vi "Plot update numeric array.vi"(8 "error in (no error)":errorcluster, 9 "Numerics":dbl[](array[numeric]), 11 "refs":T1) -> (0 "error out":errorcluster)   [LabVIEW 2021, in "RocketPlot.lvlib"]
uses:
  RocketPlot.lvlib
  TypeDefs/Plot UI references.ctl
  Classes/RocketPlotHandle/RocketPlotHandle.lvclass
  <userlib>/bjustice/TipStripOOPanel/Classes/TipPanelHandle/TipPanelHandle.lvclass
  TypeDefs/Plot top row.ctl
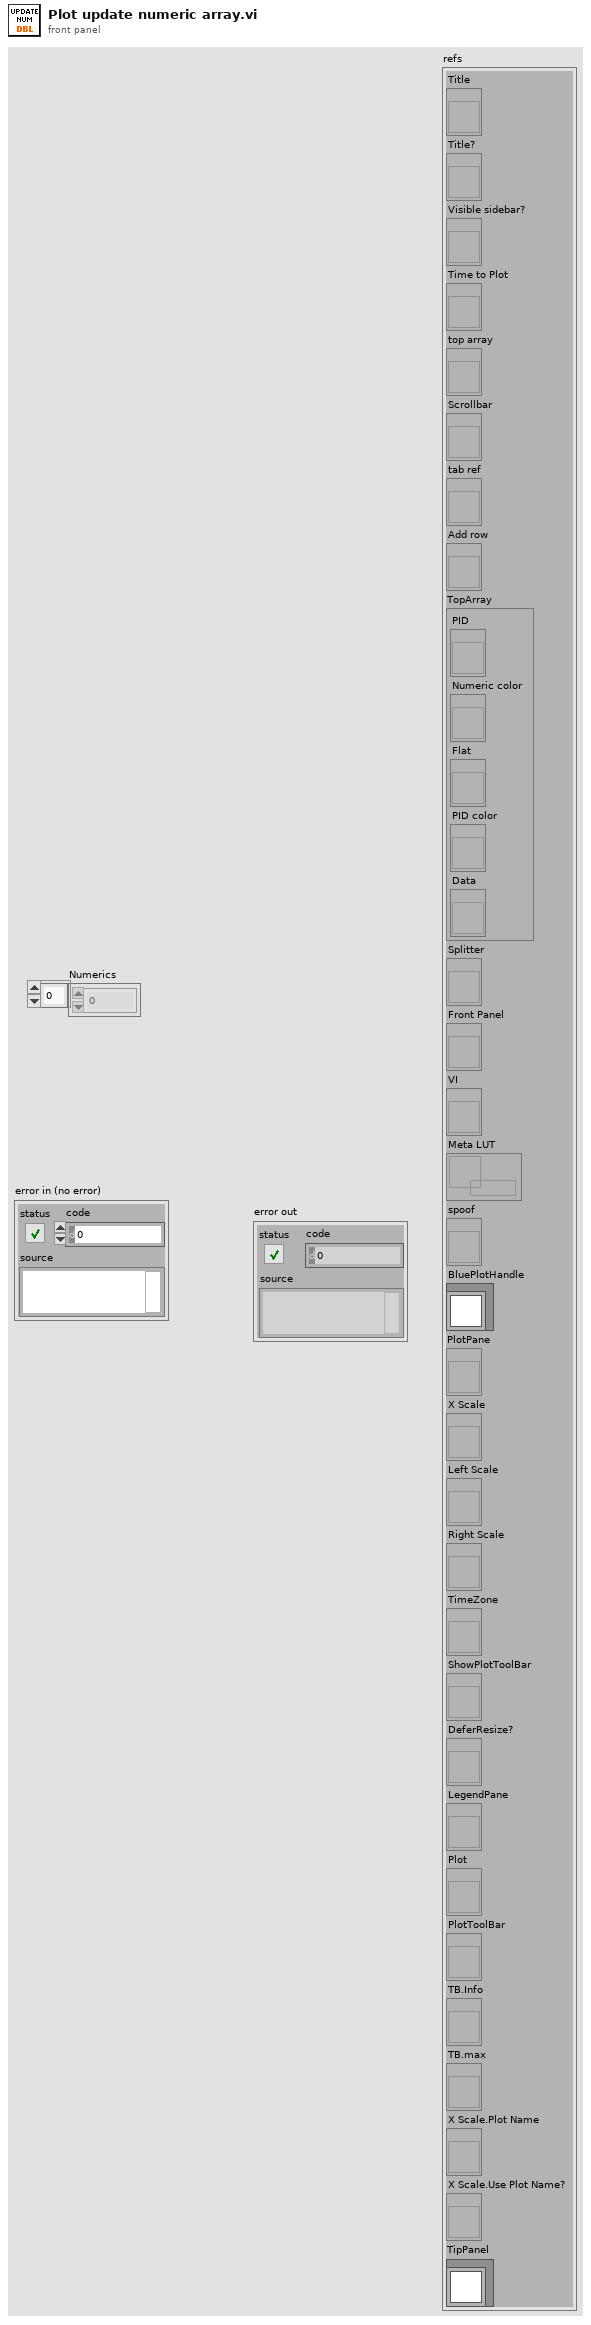
[diagram p1: front panel]
types:
  T1 = typedef "RocketPlot.lvlib/Plot UI references.ctl" = cluster{"Title":refnum<vi>, "Title?":refnum<vi>, "Visible sidebar?":refnum<vi>, "Time to Plot":refnum<vi>, "top array":refnum<vi>, "Scrollbar":refnum<vi>, "tab ref":refnum<vi>, "Add row":refnum<vi>, "TopArray":cluster{"PID":refnum<vi>, "Numeric color":refnum<vi>, "Flat":refnum<vi>, "PID color":refnum<vi>, "Data":refnum<vi>}, "Splitter":refnum<vi>, "Front Panel":refnum<vi>, "VI":refnum<vi>, "Meta LUT":refnum<data-value>, "spoof":refnum<vi>, "BluePlotHandle":refnum<class "RocketPlotHandle.lvclass">, "PlotPane":refnum<vi>, "X Scale":refnum<vi>, "Left Scale":refnum<vi>, "Right Scale":refnum<vi>, "TimeZone":refnum<vi>, "ShowPlotToolBar":refnum<vi>, "DeferResize?":refnum<vi>, "LegendPane":refnum<vi>, "Plot":refnum<vi>, "PlotToolBar":refnum<vi>, "TB.Info":refnum<vi>, "TB.max":refnum<vi>, "X Scale.Plot Name":refnum<vi>, "X Scale.Use Plot Name?":refnum<vi>, "TipPanel":refnum<class "TipPanelHandle.lvclass">}
  T2 = typedef "Plot top row.ctl" = cluster{"PID":string, "index":i32, "PID color":u32, "right axis?":bool, "Flatline?":bool, "Numeric color":u32, "Data":string, "Flat":string}
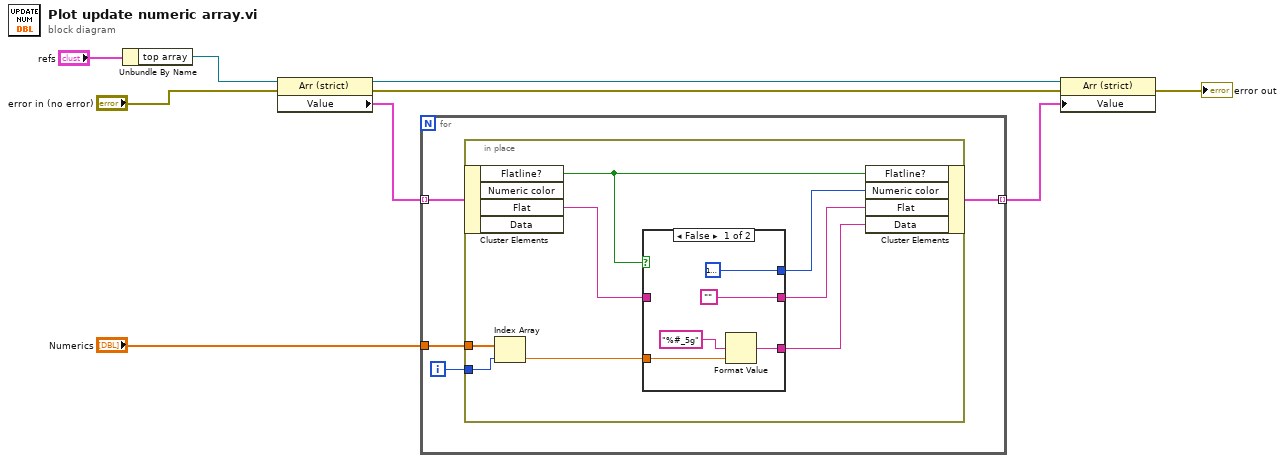
[diagram p0: block diagram]
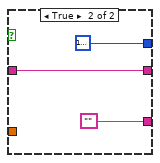
[diagram p2: hidden frame]
diagram:
  n1 = Unbundle By Name("refs") -> ("top array"=w1:refnum<vi>)
  n2 = property class="Arr (strict)"(reference=w1, error in="error in (no error)") -> (reference out=w8:refnum<vi>, error out=w7:errorcluster, "Value"=w6:T2[])
  n3 = for {
    tunnel: w6 -> [w11] mode=indexing
    tunnel: "Numerics" -> [w13]
    tunnel: [w10] -> w3 mode=indexing
    i -> [w12]
    n4 = in-place {
      in-place-border: w13 -> [w21]
      in-place-border: w12 -> [w20]
      n5 = in-place-cluster #1(w11) -> ("Flatline?"=w19:bool, "Flat"=w14:string)  [unwired: 2 out]
      n6 = Index Array(array=w21, index=w20) -> (element=w18:dbl)
      n7 = case shown="False" w19 {
        tunnel: w18 -> [w24 _]
        tunnel: [u32 16777222 u32 16777226] -> w17
        tunnel: [w23 ""] -> w15
        tunnel: ["" w27] -> w16
        tunnel: w14 -> [_ w27]
        frame False {
          n8 = Format Value(format string="%#_5g", value (0)=w24) -> (output string=w23:string)  [unwired: 1 in]
        }
        frame True {
        }
      }
      n9 = in-place-cluster #1("Flatline?"=w19, "Numeric color"=w17, "Flat"=w16, "Data"=w15) -> (w10:T2)
    }
  }
  n10 = property class="Arr (strict)"(reference=w8, error in=w7, "Value"=w3) -> (error out=→"error out":errorcluster)  [unwired: 1 out]
